vi "Helper SubVI - Online Merge PV Plot.vi"(6 "sampling rate":dbl, 7 "initialize? (F)":bool, 9 "trend  (peak:T)":bool, 10 "valley plot":cluster{"location":dbl[], "amplitude":dbl[]}[](array[cluster]), 11 "peak plot":cluster{"location":dbl[], "amplitude":dbl[]}[](array[cluster])) -> (3 "peak valley plot":cluster{"location":dbl[], "amplitude":dbl[]}[](graph))   [LabVIEW 2023]
doc: "Merges the peak plot ande valley plot."
uses:
  <vilib>/addons/_Advanced Signal Processing/NI_AdvSigProcOnlineWA.lvlib
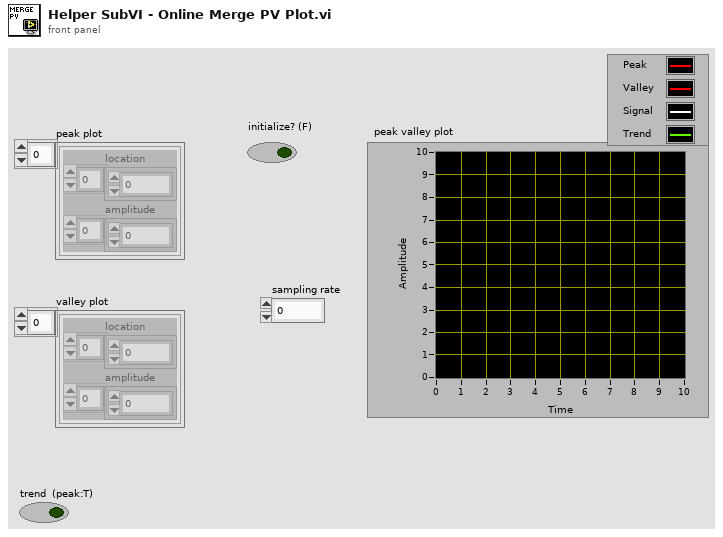
[diagram p1: front panel]
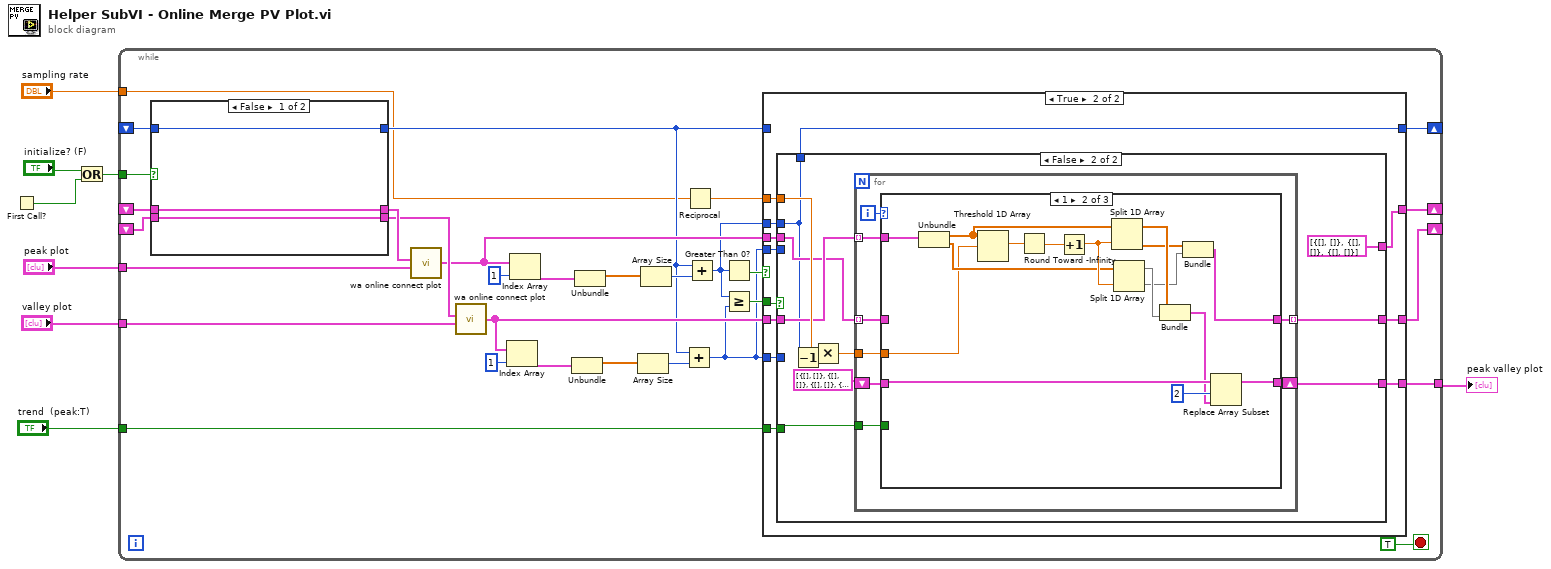
[diagram p0: block diagram]
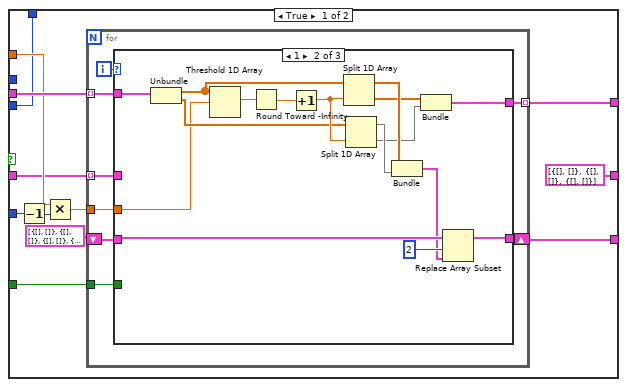
[diagram p3: hidden frame]
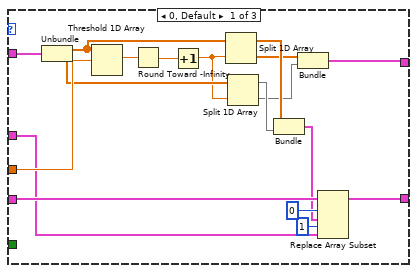
[diagram p4: hidden frame]
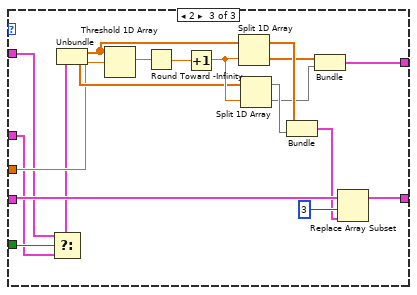
[diagram p5: hidden frame]
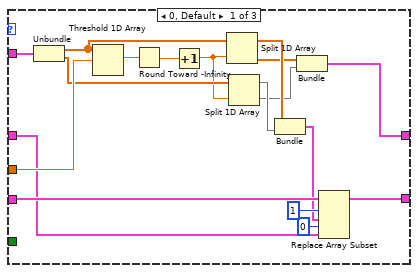
[diagram p6: hidden frame]
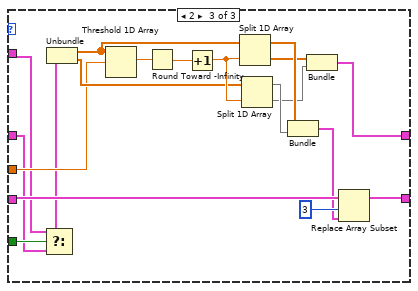
[diagram p7: hidden frame]
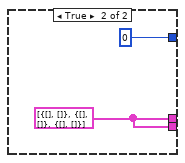
[diagram p8: hidden frame]
diagram:
  n1 = First Call?() -> (First Call?: T/F=w5:bool)
  n2 = Or(x="initialize? (F)", y=w5) -> (x .or. y?=w4:bool)
  n3 = while {
    tunnel: "peak plot" -> [w34]
    tunnel: "valley plot" -> [w32]
    tunnel: w4 -> [w39]
    shift-right: [w26] -> _
    shift-left: _ -> [w38]
    shift-right: [w24] -> _
    shift-left: _ -> [w37]
    shift-right: [w23] -> _
    shift-left: _ -> [w36]
    tunnel: [w13] -> w3
    tunnel: "sampling rate" -> [w10]
    tunnel: "trend  (peak:T)" -> [w9]
    stop <- TRUE stop-if-true
    n4 = case shown="False" w39 {
      tunnel: [w202 0] -> w17
      tunnel: w38 -> [w202 _]
      tunnel: [w201 w203] -> w35
      tunnel: [w200 w203] -> w33
      tunnel: w37 -> [w201 _]
      tunnel: w36 -> [w200 _]
      frame False {
      }
      frame True {
        w203 = cluster{"location":dbl[], "amplitude":dbl[]}[] [{"location"=[], "amplitude"=[]}, {"location"=[], "amplitude"=[]}, {"location"=[], "amplitude"=[]}] ("peak plot out")
      }
    }
    n5 = call <vilib>:"wa online connect plot.vi"("peak plot 1"=w35, "peak plot 2"=w34) -> ("peak plot out"=w25:cluster{"location":dbl[], "amplitude":dbl[]}[])  [unwired: 5 out]
    n6 = call <vilib>:"wa online connect plot.vi"("peak plot 1"=w33, "peak plot 2"=w32) -> ("peak plot out"=w18:cluster{"location":dbl[], "amplitude":dbl[]}[])  [unwired: 5 out]
    n7 = Index Array(array=w18, index=1) -> (element=w20:cluster{"location":dbl[], "amplitude":dbl[]})
    n8 = Index Array(array=w25, index=1) -> (element=w30:cluster{"location":dbl[], "amplitude":dbl[]})
    n9 = Unbundle(w20) -> ("location"=w21:dbl[])  [unwired: 1 out]
    n10 = Unbundle(w30) -> ("location"=w29:dbl[])  [unwired: 1 out]
    n11 = Array Size(array=w21) -> (size(s)=w22:i32)
    n12 = Array Size(array=w29) -> (size(s)=w28:i32)
    n13 = Add(x=w17, y=w22) -> (x+y=w11:i32)
    n14 = Reciprocal(x=w10) -> (1/x=w14:dbl)
    n15 = Add(x=w17, y=w28) -> (x+y=w12:i32)
    n16 = Greater Than 0?(x=w12) -> (x > 0?=w27:bool)
    n17 = Greater Or Equal?(x=w12, y=w11) -> (x >= y?=w16:bool)
    n18 = case shown="True" w27 {
      tunnel: w17 -> [w42 _]
      tunnel: [w42 w46] -> w26
      tunnel: w18 -> [w40 w51]
      tunnel: w25 -> [w41 w54]
      tunnel: [w41 w45] -> w24
      tunnel: [w40 w44] -> w23
      tunnel: w16 -> [_ w50]
      tunnel: w14 -> [_ w52]
      tunnel: w11 -> [_ w53]
      tunnel: [_ w49] -> w13
      tunnel: w12 -> [_ w48]
      tunnel: w11 -> [_ w47]
      tunnel: w9 -> [_ w43]
      frame False {
      }
      frame True {
        n19 = case shown="False" w50 {
          tunnel: w54 -> [w66 w132]
          tunnel: w53 -> [w65 _]
          tunnel: w52 -> [w63 w137]
          tunnel: w51 -> [w61 w133]
          tunnel: [w59 w134] -> w49
          tunnel: w48 -> [_ w128]
          tunnel: [w58 w128] -> w46
          tunnel: w47 -> [w58 _]
          tunnel: [w57 cluster{"location":dbl[], "amplitude":dbl[]}[] [{"location"=[], "amplitude"=[]}, {"location"=[], "amplitude"=[]}, {"location"=[], "amplitude"=[]}] ("peak plot out")] -> w45
          tunnel: [cluster{"location":dbl[], "amplitude":dbl[]}[] [{"location"=[], "amplitude"=[]}, {"location"=[], "amplitude"=[]}, {"location"=[], "amplitude"=[]}] ("peak plot out") w131] -> w44
          tunnel: w43 -> [w55 w129]
          frame True {
            n20 = Decrement(x=w65) -> (x-1=w64:i32)
            n21 = Multiply(x=w63, y=w64) -> (x*y=w62:dbl)
            n22 = for {
              tunnel: w66 -> [w74] mode=indexing
              tunnel: w62 -> [w73]
              tunnel: w61 -> [w71] mode=indexing
              shift-right: [w69] -> w59
              shift-left: cluster{"location":dbl[], "amplitude":dbl[]}[] [{"location"=[], "amplitude"=[]}, {"location"=[], "amplitude"=[]}, {"location"=[], "amplitude"=[]}, {"location"=[], "amplitude"=[]}] ("peak plot out") -> [w70]
              tunnel: [w68] -> w57 mode=indexing
              tunnel: w55 -> [w67]
              i -> [w72]
              n23 = case shown="1" w72 {
                tunnel: w74 -> [w92 w101 w111]
                tunnel: w73 -> [w91 w100 w120]
                tunnel: w71 -> [w79 _ w110]
                tunnel: w70 -> [w83 w99 w119]
                tunnel: [w78 w96 w116] -> w69
                tunnel: [w75 w93 w113] -> w68
                tunnel: w67 -> [_ _ w112]
                frame 0, Default {
                  n24 = Unbundle(w92) -> ("location"=w88:dbl[], "amplitude"=w87:dbl[])
                  n25 = Threshold 1D Array(2:w91, 3:w88) -> (0:w90:dbl)  [unwired: 1 out]
                  n26 = Round Toward -Infinity(1:w90) -> (0:w89:dbl)
                  n27 = Increment(x=w89) -> (x+1=w86:dbl)
                  n28 = Split 1D Array(array=w88, index=w86) -> (first subarray=w85:dbl[], second subarray=w77:dbl[])
                  n29 = Split 1D Array(array=w87, index=w86) -> (first subarray=w84:dbl[], second subarray=w76:dbl[])
                  n30 = Bundle(w85, w84) -> (w81:cluster{dbl[], dbl[]})  [unwired: 1 out]
                  n31 = Bundle(w77, w76) -> (w75:cluster{dbl[], dbl[]})  [unwired: 1 out]
                  n32 = Replace Array Subset(array=w83, new element #1=w81, index #1=0 ("index"), new element #2=w79, index #2=1 ("index")) -> (w78:cluster{"location":dbl[], "amplitude":dbl[]}[])
                }
                frame 1 {
                  n33 = Unbundle(w101) -> ("location"=w104:dbl[], "amplitude"=w105:dbl[])
                  n34 = Threshold 1D Array(2:w100, 3:w104) -> (0:w102:dbl)  [unwired: 1 out]
                  n35 = Round Toward -Infinity(1:w102) -> (0:w103:dbl)
                  n36 = Increment(x=w103) -> (x+1=w106:dbl)
                  n37 = Split 1D Array(array=w104, index=w106) -> (first subarray=w107:dbl[], second subarray=w95:dbl[])
                  n38 = Split 1D Array(array=w105, index=w106) -> (first subarray=w108:dbl[], second subarray=w94:dbl[])
                  n39 = Bundle(w107, w108) -> (w97:cluster{dbl[], dbl[]})  [unwired: 1 out]
                  n40 = Bundle(w95, w94) -> (w93:cluster{dbl[], dbl[]})  [unwired: 1 out]
                  n41 = Replace Array Subset(array=w99, new element=w97, index=2) -> (w96:cluster{"location":dbl[], "amplitude":dbl[]}[])
                }
                frame 2 {
                  n42 = Select(t=w111, s=w112, f=w110) -> (s? t:f=w109:cluster{"location":dbl[], "amplitude":dbl[]})
                  n43 = Unbundle(w109) -> ("location"=w123:dbl[], "amplitude"=w124:dbl[])
                  n44 = Threshold 1D Array(2:w120, 3:w123) -> (0:w121:dbl)  [unwired: 1 out]
                  n45 = Round Toward -Infinity(1:w121) -> (0:w122:dbl)
                  n46 = Increment(x=w122) -> (x+1=w125:dbl)
                  n47 = Split 1D Array(array=w123, index=w125) -> (first subarray=w126:dbl[], second subarray=w115:dbl[])
                  n48 = Split 1D Array(array=w124, index=w125) -> (first subarray=w127:dbl[], second subarray=w114:dbl[])
                  n49 = Bundle(w126, w127) -> (w117:cluster{dbl[], dbl[]})  [unwired: 1 out]
                  n50 = Bundle(w115, w114) -> (w113:cluster{dbl[], dbl[]})  [unwired: 1 out]
                  n51 = Replace Array Subset(array=w119, new element=w117, index=3) -> (w116:cluster{"location":dbl[], "amplitude":dbl[]}[])
                }
              }
            }
          }
          frame False {
            n52 = Decrement(x=w128) -> (x-1=w138:i32)
            n53 = Multiply(x=w137, y=w138) -> (x*y=w136:dbl)
            n54 = for {
              tunnel: w133 -> [w146] mode=indexing
              tunnel: w136 -> [w145]
              tunnel: w132 -> [w143] mode=indexing
              shift-right: [w141] -> w134
              shift-left: cluster{"location":dbl[], "amplitude":dbl[]}[] [{"location"=[], "amplitude"=[]}, {"location"=[], "amplitude"=[]}, {"location"=[], "amplitude"=[]}, {"location"=[], "amplitude"=[]}] ("peak plot out") -> [w142]
              tunnel: [w140] -> w131 mode=indexing
              tunnel: w129 -> [w139]
              i -> [w144]
              n55 = case shown="1" w144 {
                tunnel: w146 -> [w164 w173 w183]
                tunnel: w145 -> [w163 w172 w192]
                tunnel: w143 -> [w151 _ w182]
                tunnel: w142 -> [w155 w171 w191]
                tunnel: [w150 w168 w188] -> w141
                tunnel: [w147 w165 w185] -> w140
                tunnel: w139 -> [_ _ w184]
                frame 0, Default {
                  n56 = Unbundle(w164) -> ("location"=w160:dbl[], "amplitude"=w159:dbl[])
                  n57 = Threshold 1D Array(2:w163, 3:w160) -> (0:w162:dbl)  [unwired: 1 out]
                  n58 = Round Toward -Infinity(1:w162) -> (0:w161:dbl)
                  n59 = Increment(x=w161) -> (x+1=w158:dbl)
                  n60 = Split 1D Array(array=w160, index=w158) -> (first subarray=w157:dbl[], second subarray=w149:dbl[])
                  n61 = Split 1D Array(array=w159, index=w158) -> (first subarray=w156:dbl[], second subarray=w148:dbl[])
                  n62 = Bundle(w157, w156) -> (w153:cluster{dbl[], dbl[]})  [unwired: 1 out]
                  n63 = Bundle(w149, w148) -> (w147:cluster{dbl[], dbl[]})  [unwired: 1 out]
                  n64 = Replace Array Subset(array=w155, new element #1=w153, index #1=1 ("index"), new element #2=w151, index #2=0 ("index")) -> (w150:cluster{"location":dbl[], "amplitude":dbl[]}[])
                }
                frame 1 {
                  n65 = Unbundle(w173) -> ("location"=w176:dbl[], "amplitude"=w177:dbl[])
                  n66 = Threshold 1D Array(2:w172, 3:w176) -> (0:w174:dbl)  [unwired: 1 out]
                  n67 = Round Toward -Infinity(1:w174) -> (0:w175:dbl)
                  n68 = Increment(x=w175) -> (x+1=w178:dbl)
                  n69 = Split 1D Array(array=w176, index=w178) -> (first subarray=w179:dbl[], second subarray=w167:dbl[])
                  n70 = Split 1D Array(array=w177, index=w178) -> (first subarray=w180:dbl[], second subarray=w166:dbl[])
                  n71 = Bundle(w179, w180) -> (w169:cluster{dbl[], dbl[]})  [unwired: 1 out]
                  n72 = Bundle(w167, w166) -> (w165:cluster{dbl[], dbl[]})  [unwired: 1 out]
                  n73 = Replace Array Subset(array=w171, new element=w169, index=2) -> (w168:cluster{"location":dbl[], "amplitude":dbl[]}[])
                }
                frame 2 {
                  n74 = Select(t=w183, s=w184, f=w182) -> (s? t:f=w181:cluster{"location":dbl[], "amplitude":dbl[]})
                  n75 = Unbundle(w181) -> ("location"=w195:dbl[], "amplitude"=w196:dbl[])
                  n76 = Threshold 1D Array(2:w192, 3:w195) -> (0:w193:dbl)  [unwired: 1 out]
                  n77 = Round Toward -Infinity(1:w193) -> (0:w194:dbl)
                  n78 = Increment(x=w194) -> (x+1=w197:dbl)
                  n79 = Split 1D Array(array=w195, index=w197) -> (first subarray=w198:dbl[], second subarray=w187:dbl[])
                  n80 = Split 1D Array(array=w196, index=w197) -> (first subarray=w199:dbl[], second subarray=w186:dbl[])
                  n81 = Bundle(w198, w199) -> (w189:cluster{dbl[], dbl[]})  [unwired: 1 out]
                  n82 = Bundle(w187, w186) -> (w185:cluster{dbl[], dbl[]})  [unwired: 1 out]
                  n83 = Replace Array Subset(array=w191, new element=w189, index=3) -> (w188:cluster{"location":dbl[], "amplitude":dbl[]}[])
                }
              }
            }
          }
        }
      }
    }
  }
  "peak valley plot" <- w3
